vi "Format Attribute.vi"(5 "Attribute Names":string[](array[string]), 6 "Indent":i32, 7 "Attribute Values":variant[](array[variant]), 11 "IPersist in":refnum<class "IPersist.lvclass">) -> (3 "IPersist out":refnum<class "IPersist.lvclass">, 4 "Attr Strings":string[](array[string]))   [LabVIEW 2020, in "IPersist.lvlib" / "IPersist.lvclass"]
uses:
  <vilib>/gpm_packages/@cs/persistence/source/IPersist/IPersist.lvclass
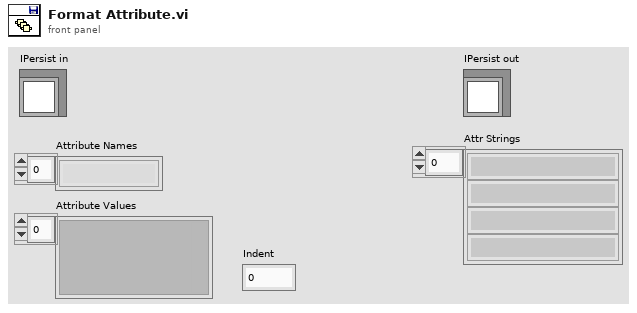
[diagram p1: front panel]
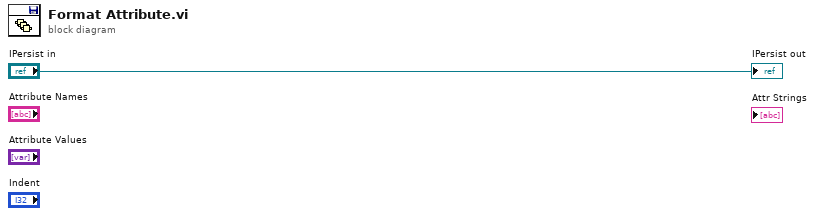
[diagram p0: block diagram]
diagram:
  "IPersist out" <- "IPersist in"
